vi "Add Test Results.vi"(8 "error in (no error)":errorcluster, 10 "Test Results":refnum<class "Test Result.lvclass">[](array[class]), 11 "ResultTree in":refnum<class "ResultTree.lvclass">) -> (0 "error out":errorcluster, 3 "ResultTree out":refnum<class "ResultTree.lvclass">)   [LabVIEW 2017, in "ResultTree.lvclass"]
doc: "Adds the specified test results to the tree."
uses:
  ResultTree.lvclass
  Test Result/Test Result.lvclass
  Test Result/Test Result.lvclass/Test Result.ctl
  Test Case/Test Case.lvclass/Test Case.ctl
  Test Result/Get Test Case.vi
  Test Result/Get Outcome.vi
  Test Case/Get Qualified Name.vi
  Test Case/Test Case.lvclass
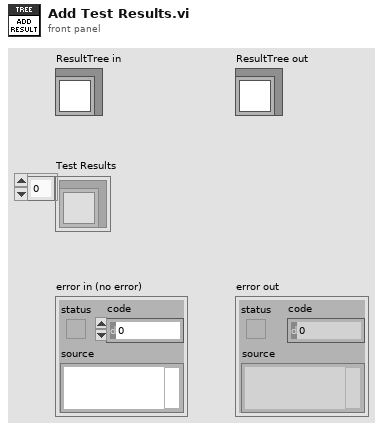
[diagram p1: front panel]
types:
  T1 = typedef "Test Outcome.ctl" = enum16{"None", "Passed", "Failed"}
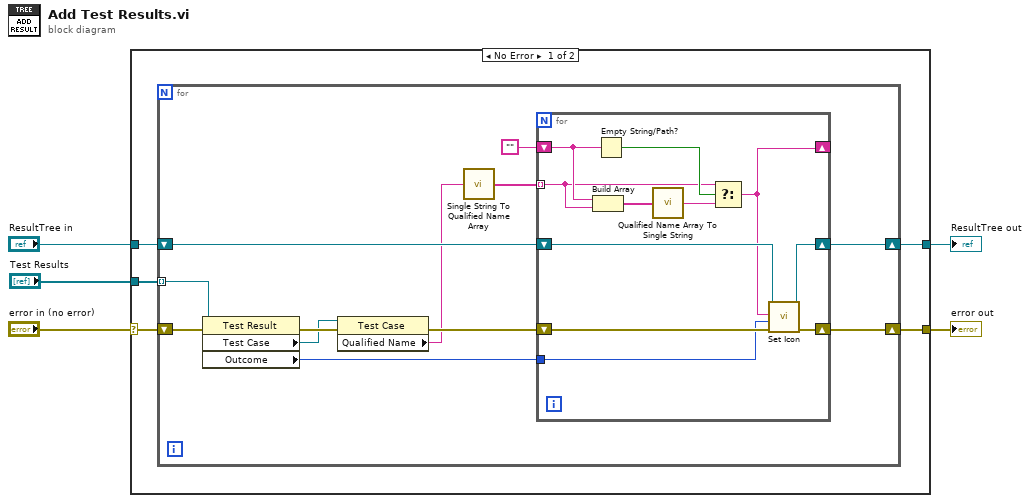
[diagram p0: block diagram]
diagram:
  n1 = case shown="No Error" "error in (no error)" {
    selector: "error in (no error)" -> [w9 w35]
    tunnel: [w10 w35] -> w4
    tunnel: [w6 w34] -> w2
    tunnel: "ResultTree in" -> [w7 w34]
    tunnel: "Test Results" -> [w8 _]
    frame No Error {
      n2 = for {
        shift-right: [w17] -> w10
        shift-left: w9 -> [w22]
        tunnel: w8 -> [w20] mode=indexing
        shift-right: [w15] -> w6
        shift-left: w7 -> [w16]
        n3 = property class="Test Result"(reference=w20, error in=w22) -> (error out=w21:errorcluster, "Test Case"=w18:refnum<class "Test Case.lvclass">, "Outcome"=w14:T1)  [unwired: 1 out]
        n4 = property class="Test Case"(reference=w18, error in=w21) -> (error out=w19:errorcluster, "Qualified Name"=w13:string)  [unwired: 1 out]
        n5 = call <vilib>:"Single String To Qualified Name Array.vi"("Fully Qualified String"=w13) -> ("Fully Qualified Array"=w12:string[])
        n6 = for {
          tunnel: w14 -> [w29]
          shift-right: [w32] -> w17
          shift-left: w19 -> [w33]
          shift-right: [w30] -> w15
          shift-left: w16 -> [w31]
          tunnel: w12 -> [w26] mode=indexing
          shift-right: [w23] -> _
          shift-left: "" -> [w27]
          n7 = Build Array(w27, w26) -> (w25:string[])
          n8 = Empty String/Path?(string/path=w27) -> (empty?=w28:bool)
          n9 = call <vilib>:"Qualified Name Array To Single String.vi"("Fully Qualified Array"=w25) -> ("Fully Qualified String"=w24:string)
          n10 = Select(t=w26, s=w28, f=w24) -> (s? t:f=w23:string)
          n11 = call "Set Icon.vi"("error in (no error)"=w33, "Icon"=w29, "Tag Name"=w23, "ResultTree in"=w31) -> ("error out"=w32:errorcluster, "ResultTree out"=w30:refnum<class "ResultTree.lvclass">)  [unwired: 6 in]
        }
      }
    }
    frame Error {
    }
  }
  "error out" <- w4
  "ResultTree out" <- w2
